vi "StartSong.vi"(8 "error in":errorcluster, 9 "Message Data":variant, 10 "Message Queues":T1, 11 "UI Refs in":T2) -> (0 "error out":errorcluster, 2 "Message Queues":T1, 3 "UI Refs out":T2, 4 "Duration":dbl)   [LabVIEW 2015]
uses:
  Controls & Type Defs/UI Data.ctl
  support/Message Queue/All Message Queues.ctl
  support/Message Queue/Message Cluster.ctl
  Controls & Type Defs/SongDetails.ctl
  support/Message Queue/Enqueue Message (Single).vi
  support/Message Queue/Message Queue.lvlib
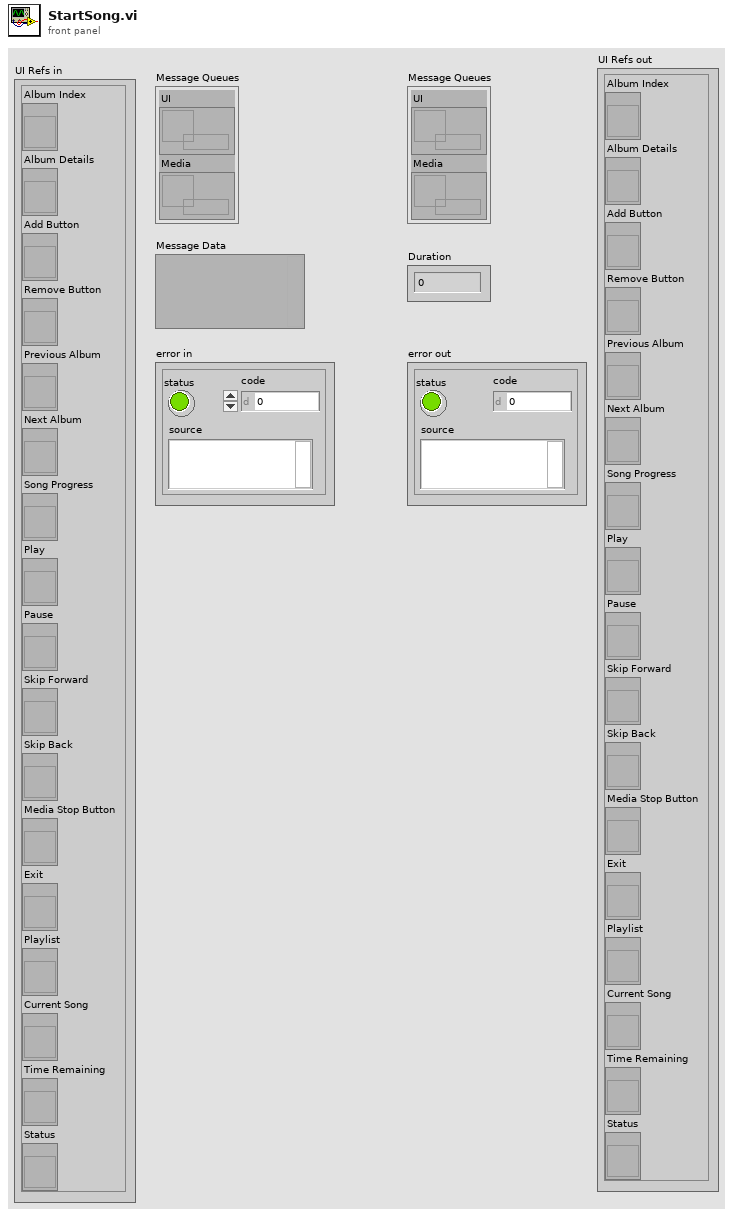
[diagram p1: front panel]
types:
  T1 = typedef "Message Queue.lvlib/All Message Queues.ctl" = cluster{"UI":refnum<queue>, "Media":refnum<queue>}
  T2 = typedef "UI Data.ctl" = cluster{"Album Index":refnum<vi>, "Album Details":refnum<vi>, "Add Button":refnum<vi>, "Remove Button":refnum<vi>, "Previous Album":refnum<vi>, "Next Album":refnum<vi>, "Song Progress":refnum<vi>, "Play":refnum<vi>, "Pause ":refnum<vi>, "Skip Forward":refnum<vi>, "Skip Back":refnum<vi>, "Media Stop Button":refnum<vi>, "Exit":refnum<vi>, "Playlist":refnum<vi>, "Current Song":refnum<vi>, "Time Remaining":refnum<vi>, "Status":refnum<vi>}
  T3 = enum8{"Enabled", "Disabled", "Disabled and Grayed Out"}
  T4 = typedef "SongDetails.ctl" = cluster{"Artist - Song Name":string, "Duration":string}
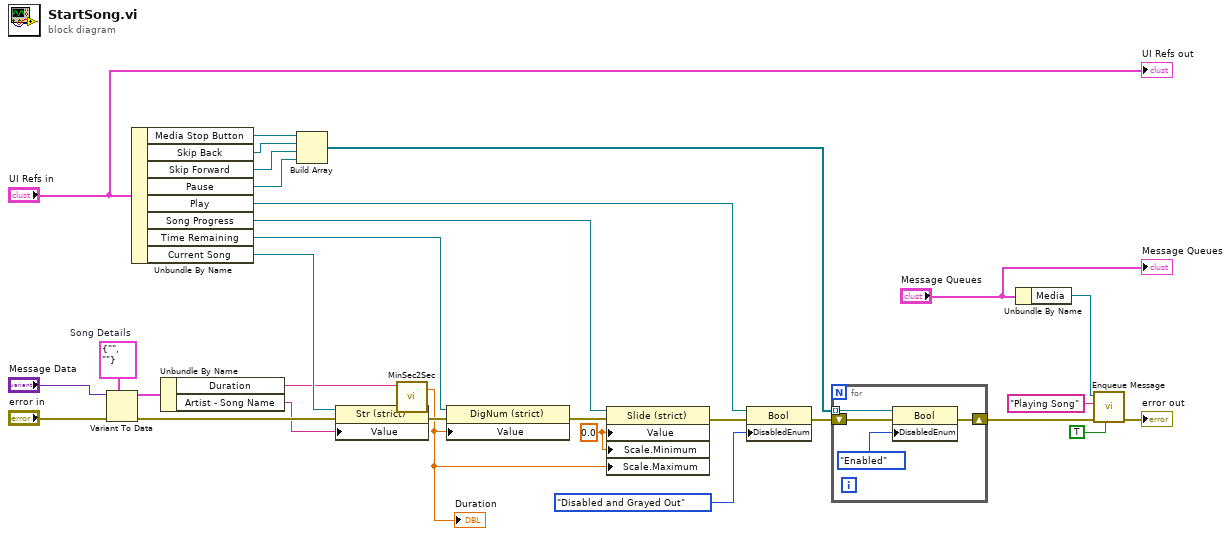
[diagram p0: block diagram]
diagram:
  w18 = 0.0 ("Value")
  w28 = T4 {"Artist - Song Name"="", "Duration"=""}  # Song Details
  n1 = Variant To Data(error in="error in", type=w28, Variant="Message Data") -> (data=w26:T4, error out=w24:errorcluster)
  n2 = Unbundle By Name("UI Refs in") -> ("Media Stop Button"=w14:refnum<vi>, "Skip Back"=w13:refnum<vi>, "Skip Forward"=w12:refnum<vi>, "Pause"=w11:refnum<vi>, "Play"=w16:refnum<vi>, "Song Progress"=w19:refnum<vi>, "Time Remaining"=w21:refnum<vi>, "Current Song"=w25:refnum<vi>)
  n3 = Unbundle By Name(w26) -> ("Duration"=w22:string, "Artist - Song Name"=w23:string)
  n4 = Build Array(w14, w13, w12, w11) -> (w9:refnum<vi>[])
  n5 = property class="Str (strict)"(reference=w25, error in=w24, "Value"=w23) -> (error out=w30:errorcluster)  [unwired: 1 out]
  n6 = call "MinSec2Sec.vi"("duration (mm:ss)"=w22) -> ("duration DBL"=w7:dbl)  [unwired: 9 in, 1 out]
  "Duration" <- w7
  n7 = property class="DigNum (strict)"(reference=w21, error in=w30, "Value"=w7) -> (error out=w20:errorcluster)  [unwired: 1 out]
  n8 = property class="Slide (strict)"(reference=w19, error in=w20, "Value"=w18, "Scale.Minimum"=w18, "Scale.Maximum"=w7) -> (error out=w17:errorcluster)  [unwired: 1 out]
  n9 = property class="Bool"(reference=w16, error in=w17, "DisabledEnum"=T3."Disabled and Grayed Out" ("Disabled")) -> (error out=w10:errorcluster)  [unwired: 1 out]
  n10 = for {
    tunnel: w9 -> [w32] mode=indexing
    shift-right: [w31] -> w6
    shift-left: w10 -> [w34]
    n11 = property class="Bool"(reference=w32, error in=w34, "DisabledEnum"=T3."Enabled" ("Disabled")) -> (error out=w31:errorcluster)  [unwired: 1 out]
  }
  n12 = Unbundle By Name("Message Queues") -> ("Media"=w3:refnum<queue>)
  n13 = call-poly "Enqueue Message.vi"("Priority Message? (F)"=TRUE, "error in (no error)"=w6, "Message"="Playing Song", "Message Queue"=w3) -> ("error out"=→"error out":errorcluster)  [unwired: 6 in, 1 out]
  "UI Refs out" <- "UI Refs in"
  "Message Queues" <- "Message Queues"
